vi "Read.vi"(8 "error in":errorcluster, 11 "Chiller Cluster - 2 Channel.lvclass":refnum<class "Cycler Cluster - 2 Channel.lvclass">) -> (0 "error out":errorcluster, 3 "output cluster":refnum<class "Cycler Cluster - 2 Channel.lvclass">)   [LabVIEW 2023, in "Cycler Cluster - 2 Channel.lvclass"]
uses:
  Cycler Cluster - 2 Channel.lvclass
  Cycler Cluster - 2 Channel.lvclass/Cycler Cluster - 2 Channel.ctl
  4448cff9-e18d-4a6b-945e-10b1e3fd2828.vi
  4a46be96-aeb5-43b7-9243-adca9a8444cf.vi
  27230f32-3038-432e-846c-8983fd03581f.vi
  4448cff9-e18d-4a6b-945e-10b1e3fd2828.vi/c28b0ead-42ad-4072-80a2-aca7f2bd7ce3.vi
  4448cff9-e18d-4a6b-945e-10b1e3fd2828.vi/219d0231-d98b-4193-b5cc-84f90e3c9091.vi
  4a46be96-aeb5-43b7-9243-adca9a8444cf.vi/c28b0ead-42ad-4072-80a2-aca7f2bd7ce3.vi
  4a46be96-aeb5-43b7-9243-adca9a8444cf.vi/219d0231-d98b-4193-b5cc-84f90e3c9091.vi
  27230f32-3038-432e-846c-8983fd03581f.vi/c28b0ead-42ad-4072-80a2-aca7f2bd7ce3.vi
  27230f32-3038-432e-846c-8983fd03581f.vi/219d0231-d98b-4193-b5cc-84f90e3c9091.vi
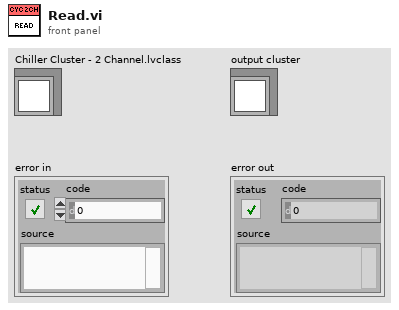
[diagram p1: front panel]
types:
  T1 = cluster{"OnOff.ACT":bool, "ErrorAcknowledge.ACT":bool, "IsoMeasurement.ACT":bool, "ParallelMode.ACT":bool}
  T2 = cluster{"ErrorAcknowledge.ch01.ACT":bool, "OutputEnable.ch01.ACT":bool, "ControlMode.ch01.CTL":u16, "Voltage.ch01.SP":dbl, "VoltageMIN.ch01.SP":dbl, "VoltageMAX.ch01.SP":dbl, "VoltageGrad.ch01.SP":dbl, "Current.ch01.SP":dbl, "CurrentMIN.ch01.SP":dbl, "CurrentMAX.ch01.SP":dbl, "CurrentGrad.ch01.SP":dbl, "Power.ch01.SP":dbl, "Power.ch01.SP":dbl, "Power.ch01.SP":dbl, "PowerGrad.ch01.SP":dbl, "ParameterSet.ch01.CTL":i32}
  T3 = cluster{"ErrorAcknowledge.ch02.ACT":bool, "OutputEnable.ch02.ACT":bool, "ControlMode.ch02.CTL":u16, "Voltage.ch02.SP":dbl, "VoltageMIN.ch02.SP":dbl, "VoltageMAX.ch02.SP":dbl, "VoltageGrad.ch02.SP":dbl, "Current.ch02.SP":dbl, "CurrentMIN.ch02.SP":dbl, "CurrentMAX.ch02.SP":dbl, "CurrentGrad.ch02.SP":dbl, "Power.ch02.SP":dbl, "PowerMIN.ch02.SP":dbl, "PowerMAX.ch02.SP":dbl, "PowerGrad.ch02.SP":dbl, "ParameterSet.ch02.CTL":i32}
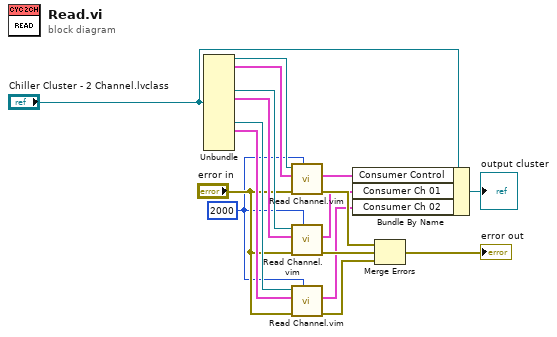
[diagram p0: block diagram]
diagram:
  w3 = 2000 ("Timeout (ms)")
  n1 = Unbundle("Chiller Cluster - 2 Channel.lvclass") -> (w16:refnum<k21>, w15:T1, w8:refnum<k21>, w7:T2, w6:refnum<k21>, w5:T3)  [unwired: 6 out]
  n2 = call "Read Channel.vim"("Timeout (ms)"=w3, "error in"="error in", "Data in"=w15, "ADAS HIL Channel in"=w16) -> ("error out"=w14:errorcluster, "Data out"=w17:T1)  [unwired: 4 in, 2 out]
  n3 = call "Read Channel.vim"("Timeout (ms)"=w3, "error in"="error in", "Data in"=w7, "ADAS HIL Channel in"=w8) -> ("error out"=w13:errorcluster, "Data out"=w9:T2)  [unwired: 4 in, 2 out]
  n4 = call "Read Channel.vim"("Timeout (ms)"=w3, "error in"="error in", "Data in"=w5, "ADAS HIL Channel in"=w6) -> ("error out"=w2:errorcluster, "Data out"=w1:T3)  [unwired: 4 in, 2 out]
  n5 = Bundle By Name(cluster="Chiller Cluster - 2 Channel.lvclass", "Consumer Control"=w17, "Consumer Ch 01"=w9, "Consumer Ch 02"=w1) -> (→"output cluster":refnum<class "Cycler Cluster - 2 Channel.lvclass">)
  n6 = Merge Errors(w14, w13, w2) -> (→"error out":errorcluster)
